vi "OutputError.vi"(8 "error in (no error)":errorcluster, 9 "Causing VI":string, 10 "Calling VI":string) -> (0 "error out":errorcluster)   [LabVIEW 2013]
doc: "Sends any errors that occur to the SmartDashboard. If the error, calling VI, and causing VI is identical to a previous error, the error will not be sent."
uses:
  <vilib>/Rock Robotics/Network Tables/SD Write Numeric Array.vi
  <vilib>/Rock Robotics/Network Tables/SD Write Boolean Array.vi
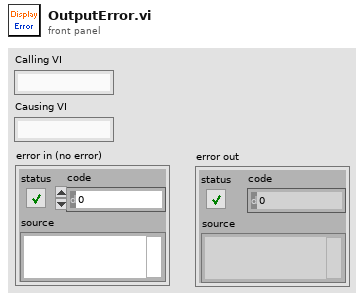
[diagram p1: front panel]
types:
  T1 = cluster{"Boolean":bool, "Numeric":i32, "String":string}
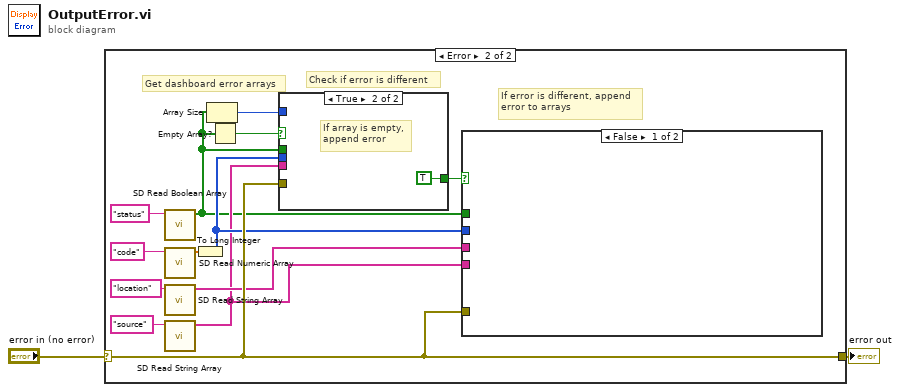
[diagram p0: block diagram]
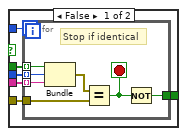
[diagram p3: hidden frame]
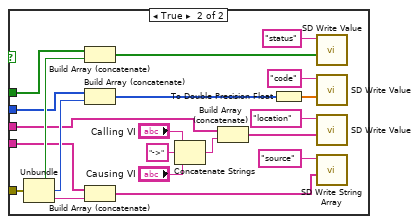
[diagram p4: hidden frame]
diagram:
  n1 = case shown="Error" "error in (no error)" {
    selector: "error in (no error)" -> [w3 w12]
    tunnel: [w3 w12] -> w1
    frame No Error {
    }
    frame Error {
      # "Check if error is different"
      # "If error is different, append\nerror to arrays"
      # "Get dashboard error arrays"
      n2 = call <vilib>:"SD Read Boolean Array.vi"("Name"="status") -> ("Boolean Array"=w5:bool[])  [unwired: 8 in, 2 out]
      n3 = call <vilib>:"SD Read Numeric Array.vi"("Name"="code") -> ("Numeric Array"=w13:dbl[])  [unwired: 8 in, 2 out]
      n4 = call <vilib>:"SD Read String Array.vi"("Name"="location") -> ("String Array"=w8:string[])  [unwired: 9 in, 1 out]
      n5 = call <vilib>:"SD Read String Array.vi"("Name"="source") -> ("String Array"=w7:string[])  [unwired: 9 in, 1 out]
      n6 = To Long Integer(number=w13) -> (32bit integer=w10:i32[])
      n7 = Array Size(array=w5) -> (size(s)=w6:i32)
      n8 = Empty Array?(array=w5) -> (empty?=w4:bool)
      n9 = case shown="True" w4 {
        tunnel: w6 -> [w22 _]
        tunnel: w12 -> [w21 _]
        tunnel: [w20 TRUE] -> w11
        tunnel: w5 -> [w19 _]
        tunnel: w10 -> [w18 _]
        tunnel: w7 -> [w17 _]
        frame False {
          n10 = for {
            N: w22 -> [_]
            tunnel: w21 -> [w26]
            tunnel: w19 -> [w29] mode=indexing
            tunnel: w18 -> [w28] mode=indexing
            tunnel: w17 -> [w27] mode=indexing
            tunnel: [w23] -> w20
            stop <- w24 stop-if-true
            # "Stop if identical"
            n11 = Bundle("Boolean"=w29, "Numeric"=w28, "String"=w27) -> (w25:T1)  [unwired: 1 in]
            n12 = Equal?(x=w25, y=w26) -> (x = y?=w24:bool)
            n13 = Not(x=w24) -> (.not. x?=w23:bool)
          }
        }
        frame True {
          # "If array is empty,\nappend error"
        }
      }
      n14 = case shown="False" w11 {
        tunnel: w12 -> [_ w51]
        tunnel: w5 -> [_ w44]
        tunnel: w10 -> [_ w41]
        tunnel: w8 -> [_ w34]
        tunnel: w7 -> [_ w35]
        frame False {
        }
        frame True {
          n15 = Unbundle(w51) -> ("status"=w43:bool, "code"=w40:i32, "source"=w36:string)
          n16 = Build Array (concatenate)(w44, w43) -> (w42:bool[])
          n17 = Build Array (concatenate)(w41, w40) -> (w39:i32[])
          n18 = Build Array (concatenate)(w35, w36) -> (w32:string[])
          n19 = Concatenate Strings("Calling VI", "->" ("string"), "Causing VI") -> (w33:string)
          n20 = Build Array (concatenate)(w34, w33) -> (w31:string[])
          n21 = To Double Precision Float(number=w39) -> (double precision float=w38:dbl[])
          n22 = call-poly <vilib>:"SD Write Value.vi"("Boolean Array"=w42, "Name"="status") -> ()  [unwired: 8 in, 2 out]
          n23 = call-poly <vilib>:"SD Write Value.vi"("Numeric Array"=w38, "Name"="code") -> ()  [unwired: 8 in, 2 out]
          n24 = call-poly <vilib>:"SD Write Value.vi"("String Array"=w31, "Name"="location") -> ()  [unwired: 8 in, 2 out]
          n25 = call <vilib>:"SD Write String Array.vi"("String Array"=w32, "Name"="source") -> ()  [unwired: 8 in, 2 out]
        }
      }
    }
  }
  "error out" <- w1
